vi "SetStageMove_Status_MotorController.vi"(8 "error in (no error)":errorcluster, 10 "Stage Moves":T1, 11 "Motor Controller in":refnum<class "Motor Controller.lvclass">) -> (0 "error out":errorcluster, 3 "Motor Controller out":refnum<class "Motor Controller.lvclass">)   [LabVIEW 2022 SP3, in "Motor Controller.lvclass"]
uses:
  Motor Controller.lvclass
  Typedefs/Stage Move Data.ctl
  Typedefs/Batch Index Speed Data.ctl
  Typedefs/Move Status.ctl
  Motor Controller.lvclass/Motor Controller.ctl
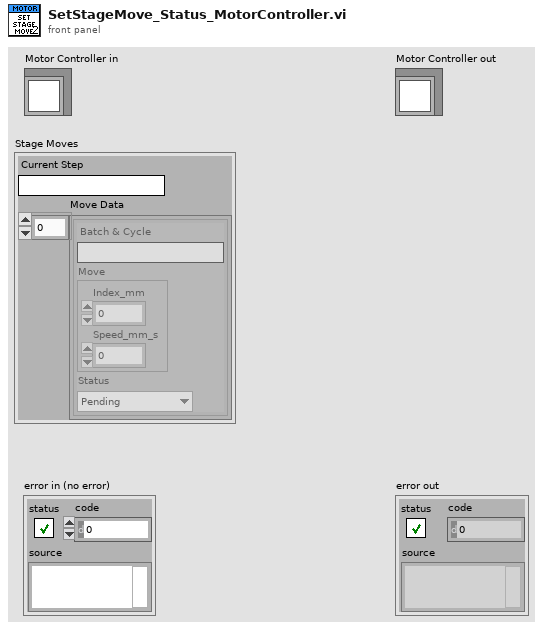
[diagram p1: front panel]
types:
  T1 = typedef "Motor Controller.lvclass/Stage Move Data.ctl" = cluster{"Current Step":string, "Move Data":T2[]}
  T2 = typedef "Motor Controller.lvclass/Batch Index Speed Data.ctl" = cluster{"Batch & Cycle":string, "Move":cluster{"Index_mm":i32, "Speed_mm_s":i32}, "Status":T3}
  T3 = typedef "Motor Controller.lvclass/Move Status.ctl" = enum16{"Pending", "In Progress", "Completed"}
  T4 = typedef "Motor Controller.lvclass/Private Data.ctl" = cluster{"UserEvents":T5, "All Dependencies":cluster{"Class References":refnum<class>[], "Class Names":string[]}, "Status":T6}
  T5 = typedef "Motor Controller.lvclass/UserEvents.ctl" = cluster{"API Incoming Event":refnum<user-event>, "API Executed Event":refnum<user-event>, "API Return Event":refnum<user-event>, "Status Changed Event":refnum<user-event>, "StopEvent":refnum<user-event>}
  T6 = typedef "Motor Controller.lvclass/Status.ctl" = cluster{"Motor Controller Config Data":T7, "Motor Controller Data":cluster{"Enabled?":bool}, "Stage Move":T1, "Stage Busy?":bool}
  T7 = typedef "Motor Controller.lvclass/Motor Controller Config Data.ctl" = cluster{"Motor IP Addresss":string, "Current Position":i32, "Pulse_Per_mm":i32, "PrePrint":dbl[], "Load Position_mm":i32, "Laminate Position_mm":i32}
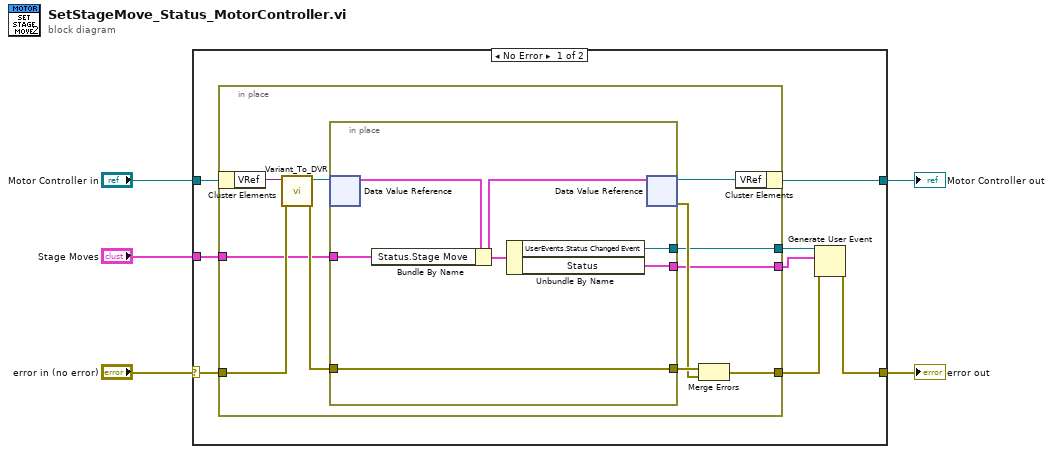
[diagram p0: block diagram]
diagram:
  n1 = case shown="No Error" "error in (no error)" {
    selector: "error in (no error)" -> [w11 w32]
    tunnel: [w7 w32] -> w2
    tunnel: [w13 w31] -> w3
    tunnel: "Motor Controller in" -> [w12 w31]
    tunnel: "Stage Moves" -> [w10 _]
    frame No Error {
      n2 = in-place {
        in-place-border: w11 -> [w22]
        in-place-border: [w18] -> w8
        in-place-border: w10 -> [w16]
        in-place-border: [w15] -> w9
        in-place-border: [w14] -> w6
        n3 = in-place-cluster #1(w12) -> ("VRef"=w24:variant)
        n4 = call "Variant_To_DVR.vi"("error in (no error)"=w22, "Variant"=w24) -> ("error out"=w21:errorcluster, "DVR"=w23:refnum<data-value>)  [unwired: 8 in]
        n5 = in-place {
          in-place-border: w21 -> [w30]
          in-place-border: [w30] -> w20
          in-place-border: w16 -> [w26]
          in-place-border: [w27] -> w15
          in-place-border: [w25] -> w14
          n6 = in-place-dvr #2(w23) -> (w29:T4)  [unwired: 1 out]
          n7 = Bundle By Name(cluster=w29, "Status.Stage Move"=w26) -> (w28:T4)
          n8 = Unbundle By Name(w28) -> ("UserEvents.Status Changed Event"=w27:refnum<user-event>, "Status"=w25:T6)
          n9 = in-place-dvr #2(w28) -> (w17:refnum<data-value>, w19:errorcluster)
        }
        n10 = Merge Errors(w20, w19) -> (w18:errorcluster)
        n11 = in-place-cluster #1("VRef"=w17) -> (w13:refnum<class "Motor Controller.lvclass">)
      }
      n12 = Generate User Event(user event=w9, event data cluster=w6, error in=w8) -> (error out=w7:errorcluster)  [unwired: 1 in, 1 out]
    }
    frame Error {
    }
  }
  "error out" <- w2
  "Motor Controller out" <- w3
